vi "Agilent VNA Read Number of Points.vi"(6 "Channel":i8=1 min=1 max=99 step=1, 7 "Agilent VNA":T1, 8 "error in (no error)":errorcluster, 11 "VISA Resource Name":refnum<visa-resource-name>) -> (0 "error out":errorcluster, 2 "Number Points":i32, 3 "dup VISA Resource Name":refnum<visa-resource-name>)   [LabVIEW 2011]
doc: "This VI for the HP 8753B is used to read the number of stimulus points."
uses:
  TypeDefs/Agilent VNA Instrument Info.ctl
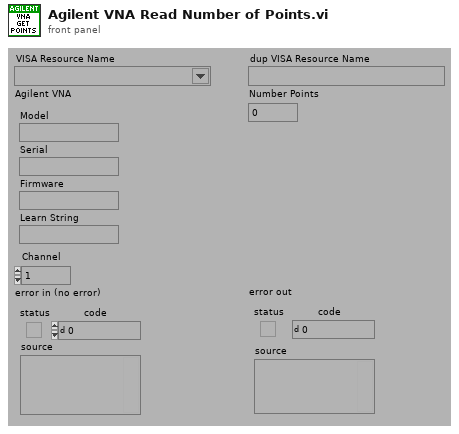
[diagram p1: front panel]
types:
  T1 = typedef "Agilent VNA Instrument Info.ctl" = cluster{"Model":string, "Serial":string, "Firmware":string, "Learn String":string}
  T2 = typedef "Agilent VNA Model.ctl" = enum16{"Not Supported", "8510X", "8719X", "8720X", "8722X", "8753X", "ENA", "PNA", "Field Fox"}
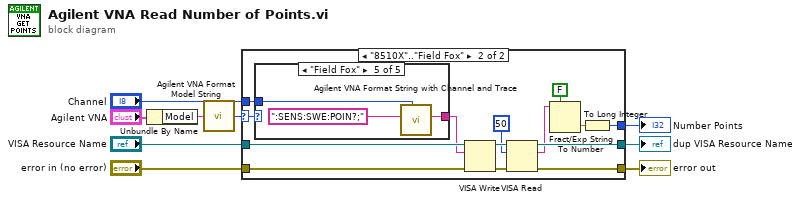
[diagram p0: block diagram]
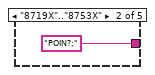
[diagram p4: hidden frame]
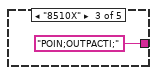
[diagram p5: hidden frame]
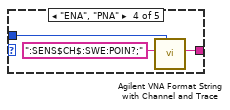
[diagram p6: hidden frame]
diagram:
  n1 = Unbundle By Name("Agilent VNA") -> ("Model"=w2:string)
  n2 = call "Agilent VNA Format Model String.vi"("Model"=w2) -> ("Model"=w1:T2)
  n3 = case shown="\"8510X\"..\"Field Fox\"" w1 {
    selector: w1 -> [_ w12]
    tunnel: [w11 w25] -> w9
    tunnel: [w10 w24] -> w8
    tunnel: "VISA Resource Name" -> [w11 w23]
    tunnel: "error in (no error)" -> [w10 w22]
    tunnel: [_ w21] -> w5
    tunnel: "Channel" -> [_ w20]
    frame "Not Supported" {
    }
    frame "8510X".."Field Fox" {
      n4 = case shown="\"Field Fox\"" w12 {
        tunnel: [_ "POIN?;" "POIN;OUTPACTI;" w29 w32] -> w13
        tunnel: w20 -> [_ _ _ w28 w31]
        frame "Not Supported" {
        }
        frame "8719X".."8753X" {
        }
        frame "8510X" {
        }
        frame "ENA", "PNA" {
          n5 = call "Agilent VNA Format String with Channel and Trace.vi"("Channel"=w28, "String"=":SENS$CH$:SWE:POIN?;") -> ("String Out"=w29:string)  [unwired: 1 in, 6 out]
        }
        frame "Field Fox" {
          n6 = call "Agilent VNA Format String with Channel and Trace.vi"("Channel"=w31, "String"=":SENS:SWE:POIN?;") -> ("String Out"=w32:string)  [unwired: 1 in, 6 out]
        }
      }
      n7 = VISA Write(VISA resource name=w23, write buffer=w13, error in (no error)=w22) -> (VISA resource name out=w16:refnum<visa-resource-name>, error out=w19:errorcluster)  [unwired: 1 out]
      n8 = VISA Read(VISA resource name=w16, byte count=u32 50, error in (no error)=w19) -> (VISA resource name out=w25:refnum<visa-resource-name>, read buffer=w18:string, error out=w24:errorcluster)  [unwired: 1 out]
      n9 = Fract/Exp String To Number(use system decimal point (T)=FALSE, string=w18) -> (number=w17:dbl)  [unwired: 3 out]
      n10 = To Long Integer(number=w17) -> (32bit integer=w21:i32)
    }
  }
  "Number Points" <- w5
  "dup VISA Resource Name" <- w9
  "error out" <- w8
